vi "update AlarmList database.vi"(8 "error in (no error)":errorcluster) -> (0 "error out":errorcluster)   [LabVIEW 2016, in "opSignIn.lvlib"]
uses:
  opSignIn.lvlib
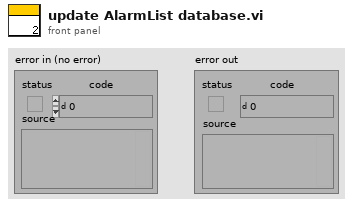
[diagram p1: front panel]
types:
  T1 = cluster{"url":string, "loginTokenRequest":cluster{"clientId":string, "clientSecret":string, "grantType":string, "password":string, "scope":string, "userName":string, "userType":string}, "自动获取MN":bool}
  T2 = cluster{"code":string, "message":string, "timestamp":u64, "data":cluster{"bearerType":string, "oauth2Type":string, "accessToken":string, "tokenType":string, "expiresIn":u64, "refreshToken":string, "scope":string[], "tokenDetail":cluster{"dataSource":string, "username":string, "userId":string, "userType":string, "enabled":bool, "accountNonExpired":bool, "credentialsNonExpired":bool, "accountNonLocked":bool}}, "success":bool}
  T3 = typedef "opSignIn.lvlib/报警格式.ctl" = cluster{"data":T4[]}
  T4 = typedef "opSignIn.lvlib/元素.ctl" = cluster{"id":string, "componentParentId":string, "componentParentName":string, "componentParentPath":string, "componentId":string, "componentName":string, "faultName":string, "equipVersion":string, "alarmCode":string, "supportAlarm":bool, "ipcAlarmCode":string, "sort":dbl, "solutionList":cluster{"id":string, "faultId":string, "reason":string, "dataPhenomenon":string, "analysis":string, "solution":string}[]}
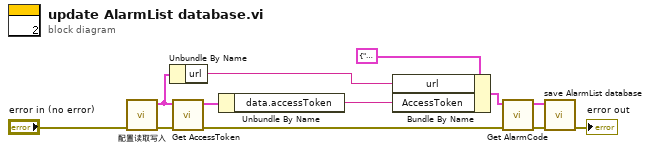
[diagram p0: block diagram]
diagram:
  n1 = call "配置读取写入.vi"("error in (no error)"="error in (no error)") -> ("error out"=w12:errorcluster, "配置输出"=w10:T1)  [unwired: 9 in]
  n2 = Unbundle By Name(w10) -> ("url"=w9:string)
  n3 = call "Get AccessToken.vi"("error in (no error)"=w12, "配置"=w10) -> ("error out"=w5:errorcluster, "response"=w8:T2)  [unwired: 8 in]
  n4 = Unbundle By Name(w8) -> ("data.accessToken"=w7:string)
  n5 = Bundle By Name(cluster=cluster{"url":string, "AccessToken":string} {"url"="http://data.watersystem.com.cn:50040", "AccessToken"="equip&GbbVkGRBUSaIfhTSjiolTAP8QMM"} ("Para"), "url"=w9, "AccessToken"=w7) -> (w6:cluster{"url":string, "AccessToken":string})
  n6 = call "Get AlarmCode.vi"("error in (no error)"=w5, "Para"=w6) -> ("error out"=w3:errorcluster, "project"=w2:T3)  [unwired: 8 in]
  n7 = call "save AlarmList database.vi"("error in (no error)"=w3, "project"=w2) -> ("error out"=→"error out":errorcluster)  [unwired: 9 in]
